vi "AddItems.vi"(6 "Shallow deps?":bool, 8 "error in (no error)":errorcluster, 9 "CDependencyQueue in":refnum<class "CDependencyQueue.lvclass">, 10 "Linker.Read Info From File":T2(array[cluster]), 11 "CDependencyInspector in":refnum<class "CDependencyInspection.lvclass">) -> (0 "error out":errorcluster, 1 "CDependencyQueue out":refnum<class "CDependencyQueue.lvclass">, 3 "CDependencyInspector out":refnum<class "CDependencyInspection.lvclass">)   [LabVIEW 2020, in "DependencyInspection.lvlib" / "CDependencyInspection.lvclass"]
uses:
  CDependencyInspection.lvclass
  <vilib>/Utility/lvfile.llb/LVFileType.ctl
  CDependencyQueue/CDependencyQueue.lvclass
  CDependencyInspection.lvclass/CDependencyInspection.ctl
  obj/Addons/LabVIEWObjectInterfaces.lvlibp/LabVIEWObjectInterfaces/ILabVIEWItem/ILabVIEWItem.lvclass
  CDebugInfo/CDebugInfo.lvclass
  CDependencyList/CDependencyList.lvclass
  obj/Addons/LabVIEWObjectFactory.lvlibp
  <vilib>/Utility/lvfile.llb/NI_FileType.lvlib
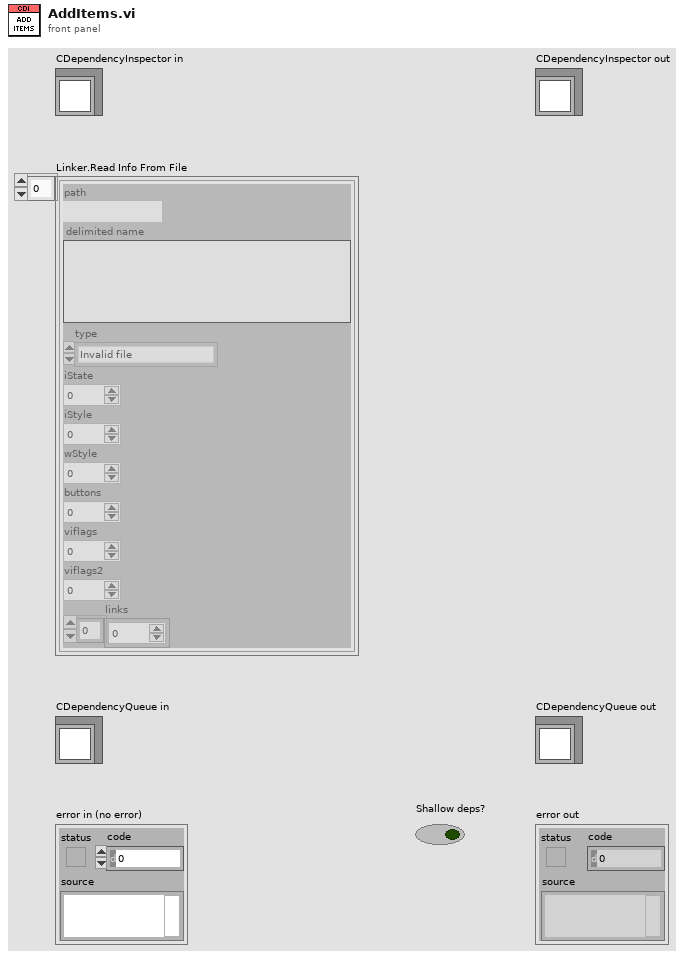
[diagram p1: front panel]
types:
  T1 = typedef "NI_FileType.lvlib/LVFileType.ctl" = enum32{"Invalid file", "Unknown type", "Instrument", "Control", "Polymorphic VI", "Project", "Library", "LVClass", "XControl", "XNode", "Shared library", ".NET assembly", "ActiveX interface", "CIN", "Run-time menu", "Palette menu", "Help file", "LLB", "XNode Edit Dependency", "Class Private Data Control", "Statechart", "MathScript .m file", "Ladder Diagram", "LVLibp", "XNode Build Dependency"}
  T2 = cluster{"path":path, "delimited name":string, "type":T1, "iState":u32, "iStyle":u16, "wStyle":u16, "buttons":u16, "viflags":u32, "viflags2":u32, "links":u32[]}[]
  T3 = cluster{"path":path, "delimited name":string, "type":T1, "iState":u32, "iStyle":u16, "wStyle":u16, "buttons":u16, "viflags":u32, "viflags2":u32, "links":u32[]}
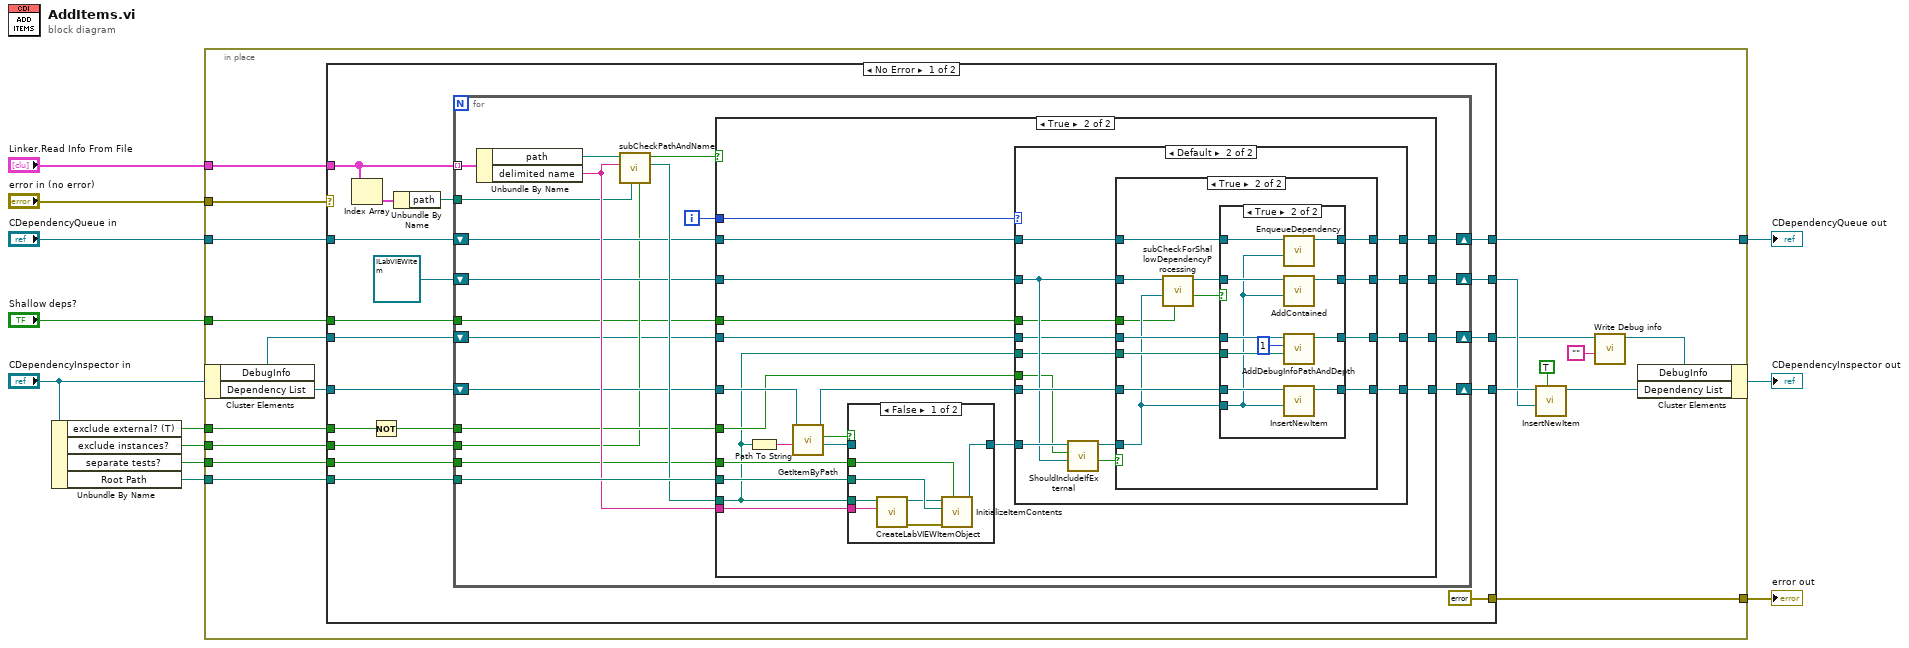
[diagram p0: block diagram]
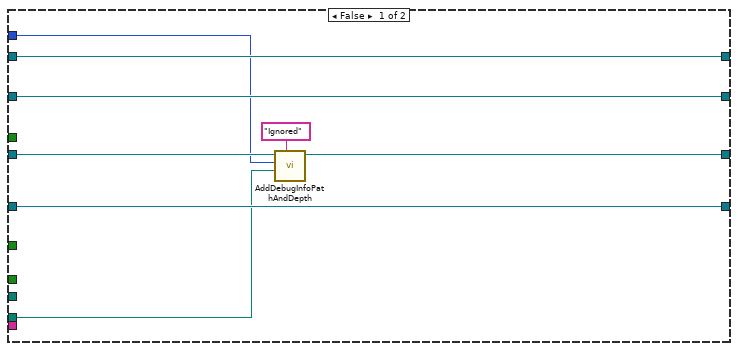
[diagram p2: hidden frame]
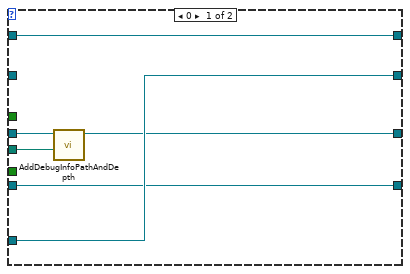
[diagram p3: hidden frame]
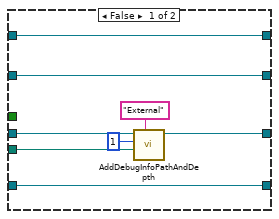
[diagram p4: hidden frame]
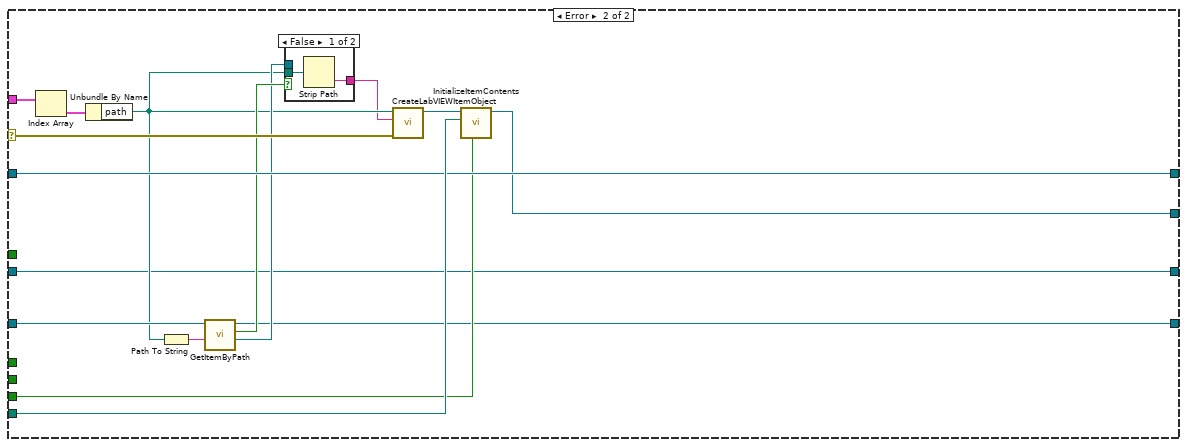
[diagram p7: hidden frame]
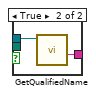
[diagram p8: hidden frame]
diagram:
  n1 = Unbundle By Name("CDependencyInspector in") -> ("exclude external? (T)"=w4:bool, "exclude instances?"=w5:bool, "separate tests?"=w6:bool, "Root Path"=w9:path)
  n2 = in-place {
    in-place-border: "error in (no error)" -> [w31]
    in-place-border: "Linker.Read Info From File" -> [w30]
    in-place-border: "CDependencyQueue in" -> [w29]
    in-place-border: w9 -> [w28]
    in-place-border: [w27] -> w8
    in-place-border: [w26] -> w7
    in-place-border: w6 -> [w25]
    in-place-border: w5 -> [w24]
    in-place-border: w4 -> [w21]
    in-place-border: "Shallow deps?" -> [w13]
    n3 = in-place-cluster #1("CDependencyInspector in") -> ("DebugInfo"=w18:refnum<class "CDebugInfo.lvclass">, "Dependency List"=w20:refnum<class "CDependencyList.lvclass">)
    n4 = case shown="No Error" w31 {
      selector: w31 -> [_ w176]
      tunnel: w30 -> [w46 w173]
      tunnel: w20 -> [w49 w170]
      tunnel: [w48 w164] -> w23
      tunnel: w28 -> [w47 w177]
      tunnel: w29 -> [w45 w175]
      tunnel: [w44 w175] -> w27
      tunnel: [errorcluster {"status"=FALSE, "code"=0, "source"=""} ("error out") _] -> w26
      tunnel: w25 -> [w40 w171]
      tunnel: w24 -> [w39 _]
      tunnel: [w37 w163] -> w17
      tunnel: w21 -> [w36 _]
      tunnel: w18 -> [w34 w162]
      tunnel: [w33 w162] -> w16
      tunnel: w13 -> [w32 _]
      frame No Error {
        n5 = Index Array(array=w46) -> (element=w43:T3)  [unwired: 1 in]
        n6 = Not(x=w36) -> (.not. x?=w35:bool)
        n7 = Unbundle By Name(w43) -> ("path"=w42:path)
        n8 = for {
          tunnel: w46 -> [w69] mode=indexing
          shift-right: [w66] -> w48
          shift-left: w49 -> [w59]
          tunnel: w47 -> [w67]
          shift-right: [w60] -> w44
          shift-left: w45 -> [w61]
          tunnel: w42 -> [w62]
          tunnel: w40 -> [w58]
          tunnel: w39 -> [w53]
          shift-right: [w57] -> w37
          shift-left: refnum<class "ILabVIEWItem.lvclass"> refnum ("ILabVIEWItem out") -> [w56]
          tunnel: w35 -> [w54]
          shift-right: [w51] -> w33
          shift-left: w34 -> [w52]
          tunnel: w32 -> [w50]
          i -> [w55]
          n9 = Unbundle By Name(w69) -> ("path"=w68:path, "delimited name"=w63:string)
          n10 = call "subCheckPathAndName.vi"("exclude instances?"=w53, "parent path"=w62, "delimited name"=w63, "path"=w68) -> ("path out"=w64:path, "path to check?"=w65:bool)  [unwired: 6 in]
          n11 = case shown="True" w65 {
            tunnel: w59 -> [w77 w94]
            tunnel: w64 -> [w72 w79]
            tunnel: w67 -> [_ w96]
            tunnel: [w77 w84] -> w66
            tunnel: w63 -> [_ w97]
            tunnel: w61 -> [w76 w87]
            tunnel: [w76 w83] -> w60
            tunnel: w58 -> [_ w95]
            tunnel: [w75 w85] -> w57
            tunnel: w56 -> [w75 w88]
            tunnel: w55 -> [w71 w90]
            tunnel: w54 -> [_ w82]
            tunnel: w52 -> [w73 w81]
            tunnel: [w74 w80] -> w51
            tunnel: w50 -> [_ w78]
            frame False {
              n12 = call-dynamic "AddDebugInfoPathAndDepth.vi"("Message"="Ignored", "Path"=w72, "Indentation"=w71, "CDebugInfo in"=w73) -> ("CDebugInfo out"=w74:refnum<class "CDebugInfo.lvclass">)  [unwired: 6 in, 1 out]
            }
            frame True {
              n13 = Path To String(path=w79) -> (string=w93:string)
              n14 = call-dynamic "GetItemByPath.vi"("Path"=w93, "CDependencyList in"=w94) -> ("ILabVIEWItem"=w92:refnum<class "ILabVIEWItem.lvclass">, "key found?"=w91:bool, "CDependencyList out"=w86:refnum<class "CDependencyList.lvclass">)  [unwired: 6 in, 1 out]
              n15 = case shown="False" w91 {
                tunnel: w97 -> [w160 _]
                tunnel: w96 -> [w159 _]
                tunnel: w95 -> [w158 _]
                tunnel: w79 -> [w157 _]
                tunnel: [w154 w161] -> w89
                tunnel: w92 -> [_ w161]
                frame False {
                  n16 = call "CreateLabVIEWItemObject.vi"("delimited name"=w160, "SubVI path"=w157) -> ("error out"=w155:errorcluster, "ILabVIEWItem"=w156:refnum<class "ILabVIEWItem.lvclass">)  [unwired: 8 in]
                  n17 = call-dynamic "InitializeItemContents.vi"("separate test?"=w158, "error in (no error)"=w155, "Root path"=w159, "ILabVIEWItem in"=w156) -> ("ILabVIEWItem out"=w154:refnum<class "ILabVIEWItem.lvclass">)  [unwired: 6 in, 1 out]
                }
                frame True {
                }
              }
              n18 = case shown="Default" w90 {
                tunnel: [w103 w113] -> w85
                tunnel: w89 -> [w103 w112]
                tunnel: w88 -> [_ w111]
                tunnel: w87 -> [w102 w117]
                tunnel: w86 -> [w101 w115]
                tunnel: [w102 w116] -> w83
                tunnel: [w101 w114] -> w84
                tunnel: w82 -> [_ w110]
                tunnel: w81 -> [w100 w107]
                tunnel: [w99 w106] -> w80
                tunnel: w79 -> [w98 w105]
                tunnel: w78 -> [_ w104]
                frame 0 {
                  n19 = call-dynamic "AddDebugInfoPathAndDepth.vi"("Path"=w98, "CDebugInfo in"=w100) -> ("CDebugInfo out"=w99:refnum<class "CDebugInfo.lvclass">)  [unwired: 8 in, 1 out]
                }
                frame Default {
                  n20 = call-dynamic "ShouldIncludeIfExternal.vi"("Current item"=w111, "Include external?"=w110, "ILabVIEWItem in"=w112) -> ("Include?"=w108:bool, "ILabVIEWItem out"=w109:refnum<class "ILabVIEWItem.lvclass">)  [unwired: 6 in, 1 out]
                  n21 = case shown="True" w108 {
                    tunnel: w117 -> [w125 w138]
                    tunnel: [w125 w126] -> w116
                    tunnel: w115 -> [w123 w137]
                    tunnel: [w123 w136] -> w114
                    tunnel: [w124 w135] -> w113
                    tunnel: w111 -> [w124 w131]
                    tunnel: w109 -> [_ w129]
                    tunnel: w107 -> [w120 w133]
                    tunnel: [w121 w134] -> w106
                    tunnel: w105 -> [w119 w132]
                    tunnel: w104 -> [_ w128]
                    frame False {
                      n22 = call-dynamic "AddDebugInfoPathAndDepth.vi"("Message"="External", "Path"=w119, "Indentation"=u8 1, "CDebugInfo in"=w120) -> ("CDebugInfo out"=w121:refnum<class "CDebugInfo.lvclass">)  [unwired: 6 in, 1 out]
                    }
                    frame True {
                      n23 = call "subCheckForShallowDependencyProcessing.vi"("Shallow deps?"=w128, "ILabVIEWItem to enqueue"=w129, "Current ILabVIEWItem in"=w131) -> ("Process?"=w127:bool, "Current ILabVIEWItem"=w130:refnum<class "ILabVIEWItem.lvclass">)  [unwired: 7 in]
                      n24 = case shown="True" w127 {
                        tunnel: w138 -> [w142 w153]
                        tunnel: w137 -> [w139 w151]
                        tunnel: [w139 w150] -> w136
                        tunnel: [w141 w149] -> w135
                        tunnel: [w140 w148] -> w134
                        tunnel: w133 -> [w140 w147]
                        tunnel: w132 -> [_ w146]
                        tunnel: w130 -> [w141 w145]
                        tunnel: w129 -> [_ w144]
                        tunnel: [w142 w152] -> w126
                        frame False {
                        }
                        frame True {
                          n25 = call-dynamic "EnqueueDependency.vi"("ILabVIEWItem to enqueue"=w144, "CDependencyQueue in"=w153) -> ("CDependencyQueue out"=w152:refnum<class "CDependencyQueue.lvclass">)  [unwired: 8 in, 1 out]
                          n26 = call-dynamic "AddContained.vi"("Item to contain"=w144, "ILabVIEWItem in"=w145) -> ("ILabVIEWItem out"=w149:refnum<class "ILabVIEWItem.lvclass">)  [unwired: 8 in, 1 out]
                          n27 = call-dynamic "AddDebugInfoPathAndDepth.vi"("Path"=w146, "Indentation"=u8 1, "CDebugInfo in"=w147) -> ("CDebugInfo out"=w148:refnum<class "CDebugInfo.lvclass">)  [unwired: 7 in, 1 out]
                          n28 = call-dynamic "InsertNewItem.vi"("ILabVIEWItem in"=w144, "CDependencyList in"=w151) -> ("CDependencyList out"=w150:refnum<class "CDependencyList.lvclass">)  [unwired: 7 in, 2 out]
                        }
                      }
                    }
                  }
                }
              }
            }
          }
        }
      }
      frame Error {
        n29 = Index Array(array=w173) -> (element=w174:T3)  [unwired: 1 in]
        n30 = Unbundle By Name(w174) -> ("path"=w166:path)
        n31 = Path To String(path=w166) -> (string=w169:string)
        n32 = call-dynamic "GetItemByPath.vi"("Path"=w169, "CDependencyList in"=w170) -> ("ILabVIEWItem"=w167:refnum<class "ILabVIEWItem.lvclass">, "key found?"=w168:bool, "CDependencyList out"=w164:refnum<class "CDependencyList.lvclass">)  [unwired: 6 in, 1 out]
        n33 = case shown="False" w168 {
          tunnel: w167 -> [_ w181]
          tunnel: w166 -> [w179 _]
          tunnel: [w178 w180] -> w165
          frame False {
            n34 = Strip Path(path=w179) -> (name=w178:string)  [unwired: 1 out]
          }
          frame True {
            n35 = call-dynamic "GetQualifiedName.vi"("ILabVIEWItem in"=w181) -> ("Qualified name"=w180:string)  [unwired: 8 in, 2 out]
          }
        }
        n36 = call "CreateLabVIEWItemObject.vi"("error in (no error)"=w176, "delimited name"=w165, "SubVI path"=w166) -> ("ILabVIEWItem"=w172:refnum<class "ILabVIEWItem.lvclass">)  [unwired: 7 in, 1 out]
        n37 = call-dynamic "InitializeItemContents.vi"("separate test?"=w171, "Root path"=w177, "ILabVIEWItem in"=w172) -> ("ILabVIEWItem out"=w163:refnum<class "ILabVIEWItem.lvclass">)  [unwired: 7 in, 1 out]
      }
    }
    n38 = call-dynamic "InsertNewItem.vi"("Replace?"=TRUE, "ILabVIEWItem in"=w17, "CDependencyList in"=w23) -> ("CDependencyList out"=w19:refnum<class "CDependencyList.lvclass">)  [unwired: 6 in, 2 out]
    n39 = call-dynamic "Write Debug info.vi"("Debug info"="", "CDebugInfo in"=w16) -> ("CDebugInfo out"=w15:refnum<class "CDebugInfo.lvclass">)  [unwired: 9 in]
    n40 = in-place-cluster #1("DebugInfo"=w15, "Dependency List"=w19) -> (→"CDependencyInspector out":refnum<class "CDependencyInspection.lvclass">)
  }
  "error out" <- w7
  "CDependencyQueue out" <- w8
